vi "Test Simple ID Query.vi"() -> ()   [LabVIEW 2023]
uses:
  EL STB Byte.ctl
  <vilib>/Instr/_visa.llb/VISA Configure Serial Port (Instr).vi
panel:
  out "read buffer":string
  out "INP STAT":string
  out "LOCK:OWN":string
  out "ERR:NEXT":string
  out "QUES":string
  out "STB Byte":T1
  out "STB":string
  out "error out":errorcluster
  out "read buffer 2":string
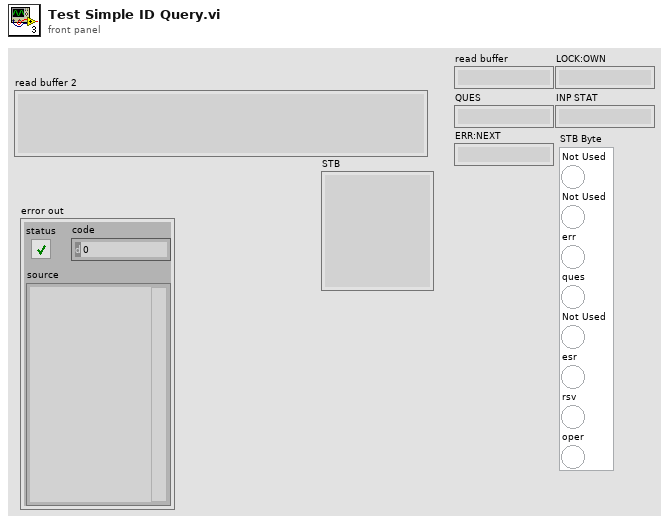
[diagram p1: front panel]
types:
  T1 = typedef "EL STB Byte.ctl" = cluster{"Not Used":bool, "Not Used":bool, "err":bool, "ques":bool, "Not Used":bool, "esr":bool, "rsv":bool, "oper":bool}
  T2 = cluster{"Boolean array[0]":bool, "Boolean array[1]":bool, "Boolean array[2]":bool, "Boolean array[3]":bool, "Boolean array[4]":bool, "Boolean array[5]":bool, "Boolean array[6]":bool, "Boolean array[7]":bool}
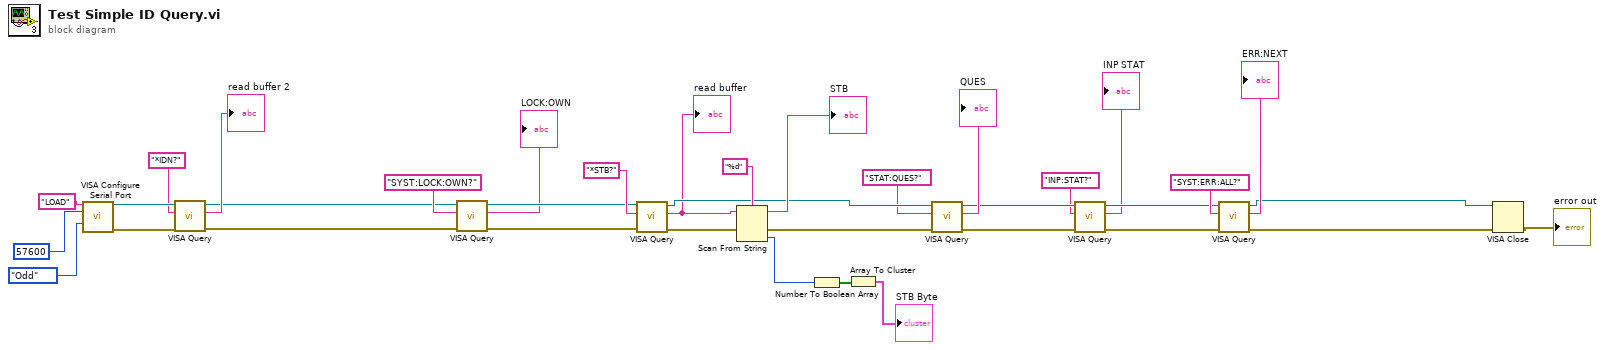
[diagram p0: block diagram]
diagram:
  n1 = call-poly "VISA Configure Serial Port"("VISA resource name"="LOAD", "baud rate (9600)"=u32 57600, "parity (0:none)"=enum16{"None", "Odd", "Even", "Mark", "Space"}."Odd") -> ("VISA resource name out"=w33:refnum<visa-resource-name>, "error out"=w30:errorcluster)  [unwired: 7 in, 4 out]
  n2 = call "VISA Query.vi"("error in (no error)"=w30, "write buffer"="*IDN?", "VISA Refnum in"=w33) -> ("error out"=w31:errorcluster, "read buffer"=→"read buffer 2":string, "VISA Refnum out"=w2:refnum<visa-resource-name>)  [unwired: 6 in]
  n3 = call "VISA Query.vi"("error in (no error)"=w31, "write buffer"="SYST:LOCK:OWN?", "VISA Refnum in"=w2) -> ("error out"=w13:errorcluster, "read buffer"=→"LOCK:OWN":string, "VISA Refnum out"=w12:refnum<visa-resource-name>)  [unwired: 6 in]
  n4 = call "VISA Query.vi"("error in (no error)"=w13, "write buffer"="*STB?", "VISA Refnum in"=w12) -> ("error out"=w27:errorcluster, "read buffer"=w1:string, "VISA Refnum out"=w19:refnum<visa-resource-name>)  [unwired: 6 in]
  "read buffer" <- w1
  n5 = Scan From String(format string="%d", input string=w1, error in=w27) -> (remaining string=→"STB":string, error out=w26:errorcluster, output 1=w23:i32)  [unwired: 2 in, 1 out]
  n6 = Number To Boolean Array(number=w23) -> (Boolean array=w22:bool[])
  n7 = Array To Cluster(array=w22) -> (cluster=→"STB Byte":T2)
  n8 = call "VISA Query.vi"("error in (no error)"=w26, "write buffer"="STAT:QUES?", "VISA Refnum in"=w19) -> ("error out"=w20:errorcluster, "read buffer"=→"QUES":string, "VISA Refnum out"=w6:refnum<visa-resource-name>)  [unwired: 6 in]
  n9 = call "VISA Query.vi"("error in (no error)"=w20, "write buffer"="INP:STAT?", "VISA Refnum in"=w6) -> ("error out"=w7:errorcluster, "read buffer"=→"INP STAT":string, "VISA Refnum out"=w5:refnum<visa-resource-name>)  [unwired: 6 in]
  n10 = call "VISA Query.vi"("error in (no error)"=w7, "write buffer"="SYST:ERR:ALL?", "VISA Refnum in"=w5) -> ("error out"=w8:errorcluster, "read buffer"=→"ERR:NEXT":string, "VISA Refnum out"=w9:refnum<visa-resource-name>)  [unwired: 6 in]
  n11 = VISA Close(VISA resource name=w9, error in (no error)=w8) -> (error out=→"error out":errorcluster)
